vi "Open Hardware.vi"(8 "error in (no error)":errorcluster, 11 "Inst.TC in":refnum<class "Inst.TC.lvclass">) -> (0 "error out":errorcluster, 3 "Inst.TC out":refnum<class "Inst.TC.lvclass">)   [LabVIEW 2019, in "Inst.TC.lvclass"]
uses:
  Inst.TC.lvclass
  <userlib>/LevyLab/Instrument Framework/Instrument Types/Cryostat/Instrument.Cryostat.lvclass
  <userlib>/LevyLab/Instrument Framework/Instrument/Instrument.lvclass
  C:/Program Files (x86)/National Instruments/LabVIEW 2019/user.lib/LevyLab/Instrument Framework/Instrument/Instrument.lvclass
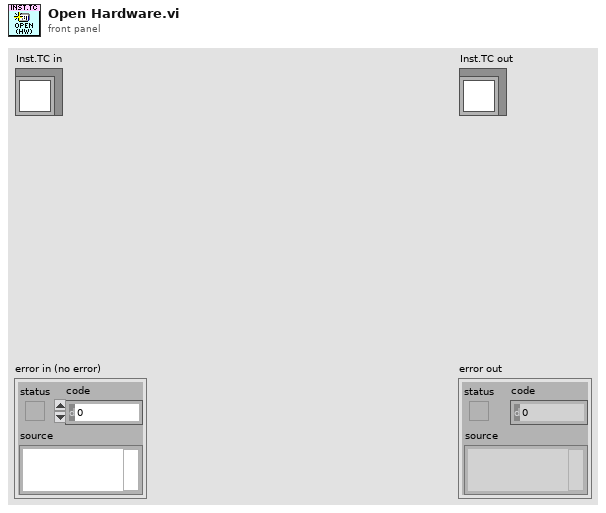
[diagram p1: front panel]
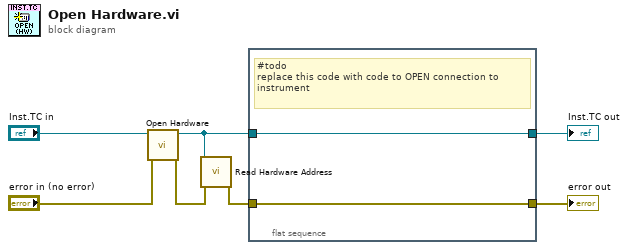
[diagram p0: block diagram]
diagram:
  n1 = call-parent "Open Hardware.vi"("error in (no error)"="error in (no error)", "Instrument in"="Inst.TC in") -> ("error out"=w5:errorcluster, "Instrument out"=w4:refnum<class "Inst.TC.lvclass">)  [unwired: 8 in]
  n2 = call <userlib>:"Read Hardware Address.vi"("error in (no error)"=w5, "Instrument in"=w4) -> ("error out"=w2:errorcluster)  [unwired: 7 in, 2 out]
  n3 = flat-sequence {
    tunnel: w4 -> [w8]
    tunnel: [w8] -> w3
    tunnel: w2 -> [w9]
    tunnel: [w9] -> w1
    frame #0 {
      # "#todo\nreplace this code with code to OPEN connection to instrument"
    }
  }
  "error out" <- w1
  "Inst.TC out" <- w3
